vi "send_GapFree-v02.vi"(0 "daq_ao 2":tag="Dev1/ao1", 1 "Duration (s)":dbl, 2 "controls array in":refnum<vi>[](array[refnum]), 3 "Sample Freq (Hz)":dbl min=0.0 max=40000.0, 6 "daq_ai":tag="Dev1/ai0:1", 9 "Number of Replicates":i16=1 min=1 max=10, 13 "error in":errorcluster) -> (12 "experiment cmd VI ref":refnum<vi>, 14 "output cluster":T1, 16 "control array out":refnum<vi>[](array[refnum]), 18 "error out":errorcluster, 19 "jumptestMonitor":waveform(dbl)[](graph))   [LabVIEW 2019]
uses:
  <vilib>/measure/NI_MABase.lvlib
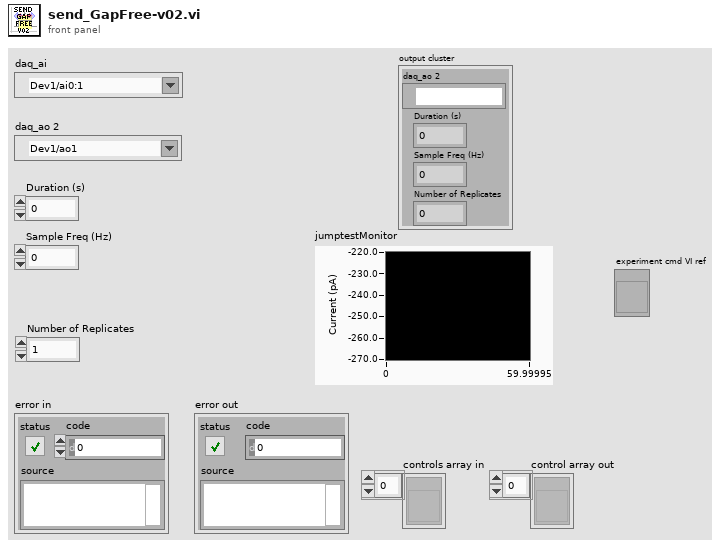
[diagram p1: front panel]
types:
  T1 = cluster{"daq_ao 2":tag, "Duration (s)":dbl, "Sample Freq (Hz)":dbl, "Number of Replicates":i16}
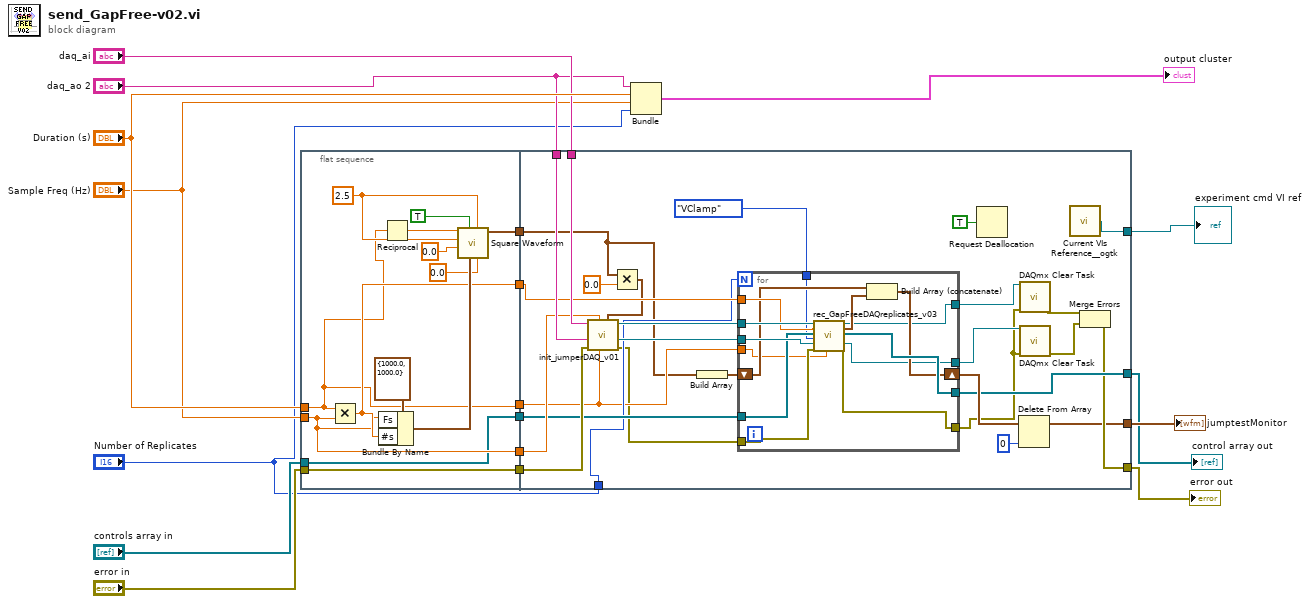
[diagram p0: block diagram]
diagram:
  n1 = flat-sequence {
    tunnel: "Duration (s)" -> [w21]
    tunnel: "Sample Freq (Hz)" -> [w26]
    tunnel: [w27] -> w13
    tunnel: [w26] -> w11
    tunnel: [w25] -> w12
    tunnel: "error in" -> [w23]
    tunnel: [w23] -> w9
    tunnel: "controls array in" -> [w22]
    tunnel: [w22] -> w7
    tunnel: [w21] -> w4
    tunnel: w13 -> [w53]
    tunnel: w12 -> [w35]
    tunnel: "daq_ai" -> [w57]
    tunnel: "daq_ao 2" -> [w56]
    tunnel: w11 -> [w55]
    tunnel: [w39] -> w15
    tunnel: "Number of Replicates" -> [w47]
    tunnel: w9 -> [w50]
    tunnel: [w42] -> w8
    tunnel: w7 -> [w49]
    tunnel: [w48] -> w6
    tunnel: w4 -> [w37]
    tunnel: [w34] -> w1
    frame #0 {
      w31 = 2.5 ("Amplitude")
      n2 = Multiply(x=w21, y=w26) -> (x*y=w27:dbl)
      n3 = Bundle By Name(cluster=cluster{"Fs":dbl, "#s":dbl} {"Fs"=1000.0, "#s"=1000.0} ("sampling info"), "Fs"=w26, "#s"=w27) -> (w28:cluster{"Fs":dbl, "#s":dbl})
      n4 = Reciprocal(x=w21) -> (1/x=w24:dbl)
      n5 = call <vilib>:"Square Waveform.vi"("duty cycle (%)"=0.0, "offset"=w31, "sampling info"=w28, "reset signal"=TRUE, "phase"=0.0, "amplitude"=w31, "frequency"=w24) -> ("signal out"=w25:waveform(dbl))  [unwired: 3 in, 1 out]
    }
    frame #1 {
      n6 = Multiply(x=w35, y=0.0) -> (x*y=w51:waveform(dbl))
      n7 = call "init_jumperDAQ_v01.vi"("protocol waveform"=w51, "Duration (s)"=w37, "Sample Freq (Hz)"=w55, "AO error in"=w50, "AO physical channels"=w56, "AI Physical Channel"=w57) -> ("AO error out"=w36:errorcluster, "AO task out"=w59:refnum<k21>, "AI task out"=w58:refnum<k21>)  [unwired: 1 in, 2 out]
      n8 = Build Array(w35) -> (w40:waveform(dbl)[])
      n9 = for {
        N: w47 -> [_]
        tunnel: w59 -> [w72]
        tunnel: w58 -> [w71]
        tunnel: w53 -> [w69]
        tunnel: w49 -> [w68]
        tunnel: [w67] -> w48
        shift-right: [w65] -> w54
        shift-left: w40 -> [w64]
        tunnel: w36 -> [w73]
        tunnel: [w70] -> w44
        tunnel: [w63] -> w46
        tunnel: [w62] -> w45
        tunnel: w37 -> [w61]
        tunnel: enum16{"VClamp", "IClamp"}."VClamp" ("which clamp") -> [w60]
        n10 = call "rec_GapFreeDAQreplicates_v03.vi"("AI task in"=w71, "number of samples"=w69, "controls array in"=w68, "which clamp"=w60, "AO task in"=w72, "error in"=w73, "Duration (s)"=w61) -> ("AI task out"=w63:refnum<k21>, "data out (pA or mV)"=w66:waveform(dbl), "control array out"=w67:refnum<vi>[], "AO task out"=w62:refnum<k21>, "error out"=w70:errorcluster)  [unwired: 8 in]
        n11 = Build Array (concatenate)(w64, w66) -> (w65:waveform(dbl)[])
      }
      n12 = Request Deallocation(TRUE ("flag")) -> ()
      n13 = Delete From Array(array=w54, index=0) -> (array with subset deleted=w39:waveform(dbl)[])  [unwired: 1 in, 1 out]
      n14 = call <vilib>:"DAQmx Clear Task.vi"("task in"=w46, "error in"=w44) -> ("error out"=w43:errorcluster)  [unwired: 13 in]
      n15 = call <vilib>:"DAQmx Clear Task.vi"("task in"=w45, "error in"=w44) -> ("error out"=w41:errorcluster)  [unwired: 13 in]
      n16 = call "Current VIs Reference__ogtk.vi"() -> ("Current VI's reference"=w34:refnum<vi>)  [unwired: 5 in]
      n17 = Merge Errors(w43, w41) -> (w42:errorcluster)
    }
  }
  n18 = Bundle("daq_ao 2"="daq_ao 2", "Duration (s)"="Duration (s)", "Sample Freq (Hz)"="Sample Freq (Hz)", "Number of Replicates"="Number of Replicates") -> (→"output cluster":T1)  [unwired: 1 in]
  "jumptestMonitor" <- w15
  "error out" <- w8
  "control array out" <- w6
  "experiment cmd VI ref" <- w1
